vi "CurrentLevelGlobal.vi"() -> ()   [LabVIEW 2018]
panel:
  out "CurrentLevelGlobal":dbl
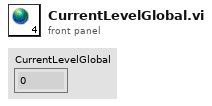
[diagram p1: front panel]
diagram:
